vi "INI read LO sharing.vi"(8 "error in (no error)":T2) -> (0 "error out":T2, 3 "data":T1)   [LabVIEW 2019, in "Shared.lvlib"]
doc: "Read mmWave LOs to export"
uses:
  Shared.lvlib
  mmWave HW Control/LO export.ctl
  Low-level/TypeDefs/TX trigger config.ctl
  FPGA/SubVIs/Utility/FPGA driver trigger source.ctl
  FPGA/SubVIs/Utility/FPGA driver trigger destination.ctl
  System GV.vi
  <vilib>/Utility/config.llb/NI_LVConfig.lvlib
  FPGA/SubVIs/Utility/FPGA Utility.lvlib
  mmWave HW Control/mmWave HW Control.lvlib
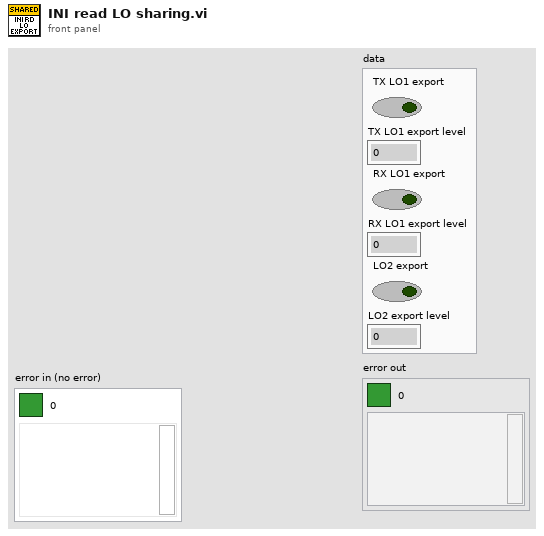
[diagram p1: front panel]
types:
  T1 = typedef "mmWave HW Control.lvlib/LO export.ctl" = cluster{"TX LO1 export":bool, "TX LO1 export level":dbl, "RX LO1 export":bool, "RX LO1 export level":dbl, "LO2 export":bool, "LO2 export level":dbl}
  T2 = cluster{"Boolean Round":bool, "code":i32, "source":string}
  T3 = typedef "TX trigger config.ctl" = cluster{"delay":dbl, "trig source":T4, "PXI src":i32, "export":T5, "PXI dest":i32}
  T4 = typedef "FPGA Utility.lvlib/FPGA driver trigger source.ctl" = enum16{"Use Tclk", "PXI_Trig", "Aurora RX trig"}
  T5 = typedef "FPGA Utility.lvlib/FPGA driver trigger destination.ctl" = enum16{"None", "Source trig", "Synced trig", "Delayed sync"}
  T6 = typedef "NI_LVConfig.lvlib/Config Data RefNum.ctl" = refnum<k1>
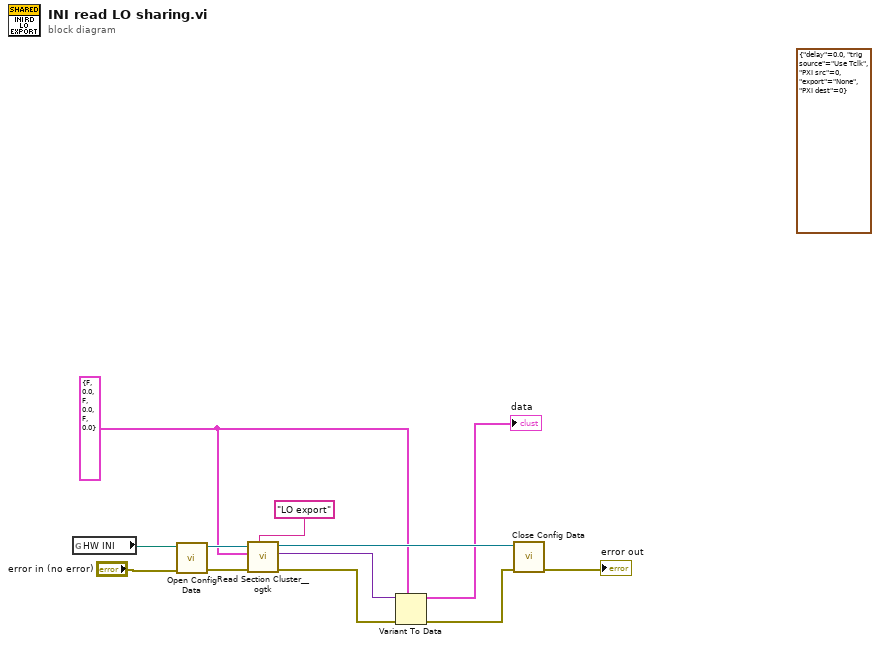
[diagram p0: block diagram]
diagram:
  w2 = T1 {"TX LO1 export"=FALSE, "TX LO1 export level"=0.0, "RX LO1 export"=FALSE, "RX LO1 export level"=0.0, "LO2 export"=FALSE, "LO2 export level"=0.0} ("LO Export")
  (unwired) T3 {"delay"=0.0, "trig source"=enum."Use Tclk", "PXI src"=0, "export"=enum."None", "PXI dest"=0} ("TX trigger options")
  n1 = global read "System GV.vi" "HW INI"() -> (w9:path)
  n2 = call <vilib>:"Open Config Data.vi"("error in (no error)"="error in (no error)", "configuration file path"=w9) -> ("error out"=w10:errorcluster, "refnum"=w12:T6)  [unwired: 7 in, 1 out]
  n3 = call <userlib>:"Read Section Cluster__ogtk.vi"("section (optional)"="LO export", "error in (no error)"=w10, "Section Formatted Cluster Type"=w2, "refnum"=w12) -> ("error out"=w6:errorcluster, "Section Formatted Cluster"=w7:variant, "dup refnum"=w11:T6)  [unwired: 3 in, 2 out]
  n4 = Variant To Data(error in=w6, type=w2, Variant=w7) -> (data=→"data":T1, error out=w5:errorcluster)
  n5 = call <vilib>:"Close Config Data.vi"("error in (no error)"=w5, "refnum"=w11) -> ("error out"=→"error out":errorcluster)  [unwired: 8 in, 1 out]
